vi "Delete FITS.vi"(8 "error in (no error)":errorcluster, 11 "Save Image in":refnum<class "Save Image.lvclass">) -> (0 "error out":errorcluster, 3 "Save Image out":refnum<class "Save Image.lvclass">)   [LabVIEW 2018, in "Save Image.lvclass"]
uses:
  Save Image.lvclass
  Simulated_Header/Simulated_Header.lvclass
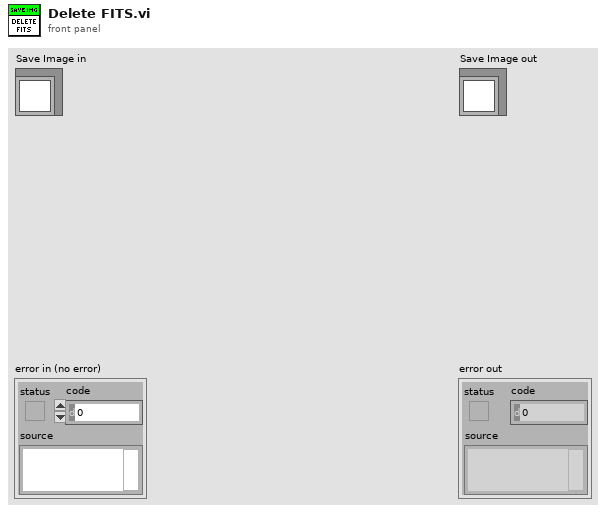
[diagram p1: front panel]
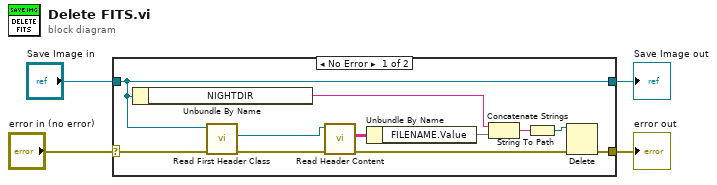
[diagram p0: block diagram]
diagram:
  n1 = case shown="No Error" "error in (no error)" {
    selector: "error in (no error)" -> [w14 w17]
    tunnel: [w15 w17] -> w3
    tunnel: [w5 w16] -> w1
    tunnel: "Save Image in" -> [w5 w16]
    frame No Error {
      n2 = Unbundle By Name(w5) -> ("NIGHTDIR"=w10:string)
      n3 = call "Read First Header Class.vi"("error in (no error)"=w14, "Save Image in"=w5) -> ("error out"=w12:errorcluster, "Simulated_Header.lvclass"=w13:refnum<class "Simulated_Header.lvclass">)  [unwired: 7 in, 1 out]
      n4 = call "Read Header Content.vi"("error in (no error)"=w12, "Simulated_Header in"=w13) -> ("error out"=w6:errorcluster, "Header Content"=w11:string[][])  [unwired: 7 in, 1 out]
      n5 = Unbundle By Name(w11) -> ("FILENAME.Value"=w9)
      n6 = Concatenate Strings(w10, w9) -> (w8:string)
      n7 = String To Path(string=w8) -> (path=w7:path)
      n8 = Delete(path (use dialog)=w7, error in=w6) -> (error out=w15:errorcluster)  [unwired: 3 in, 2 out]
    }
    frame Error {
    }
  }
  "error out" <- w3
  "Save Image out" <- w1
